vi "Write UserPwd DB Obj.vi"(10 "UserPwd DB.lvlib:UserPwd DB.lvclass":refnum<class "UserPwd DB.lvclass">, 11 "UserPwd DB Configuration in":refnum<class "UserPwd DB Configuration.lvclass">) -> (3 "UserPwd DB Configuration out":refnum<class "UserPwd DB Configuration.lvclass">)   [LabVIEW 2016, in "UserPwd DB.lvlib" / "UserPwd DB Configuration.lvclass"]
uses:
  <userlib>/Common Components/UserPwd DB/UserPwd DB Config/UserPwd DB Configuration.lvclass
  <userlib>/Common Components/UserPwd DB/UserPwd DB/UserPwd DB.lvclass
  <userlib>/Common Components/UserPwd DB/UserPwd DB Config/UserPwd DB Configuration.lvclass/UserPwd DB Configuration.ctl
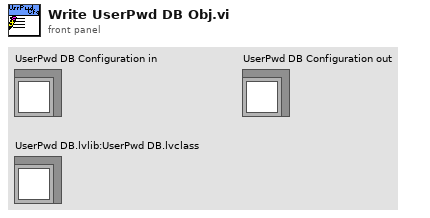
[diagram p1: front panel]
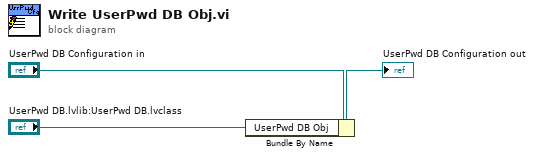
[diagram p0: block diagram]
diagram:
  n1 = Bundle By Name(cluster="UserPwd DB Configuration in", "UserPwd DB Obj"="UserPwd DB.lvlib:UserPwd DB.lvclass") -> (→"UserPwd DB Configuration out":refnum<class "UserPwd DB Configuration.lvclass">)
